vi "FV-resample-split_water.vi"(5 "Max Frequency":dbl, 7 "min Frequency":dbl, 10 "water":T1) -> (2 "water out":T1)   [LabVIEW 2020, in "FV-file_viewer.lvlib"]
uses:
  FV-file_viewer.lvlib
  FV-water_cluster.ctl
  FV-single_XY_plot.ctl
panel:
  out "Position":i32
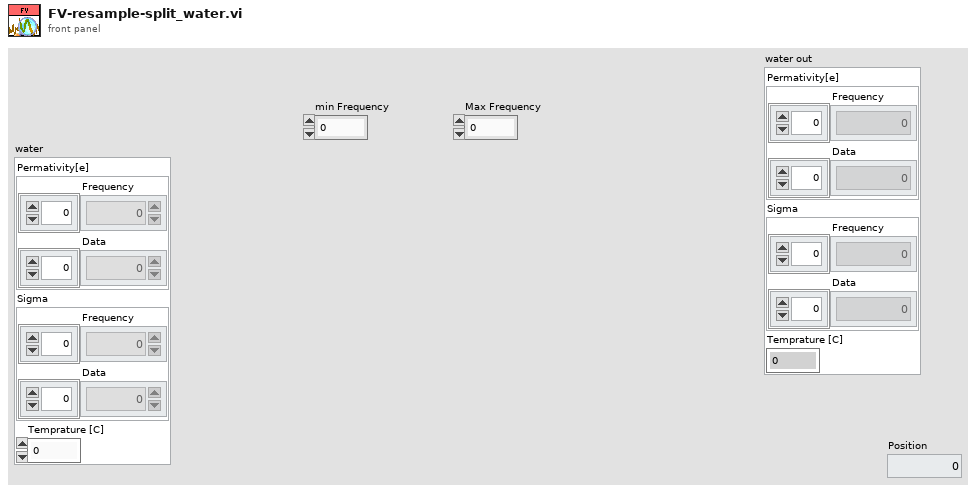
[diagram p1: front panel]
types:
  T1 = typedef "FV-file_viewer.lvlib/FV-water_cluster.ctl" = cluster{"Permativity[e]":T2, "Sigma":T2, "Temprature [C]":dbl}
  T2 = typedef "FV-file_viewer.lvlib/FV-single_XY_plot.ctl" = cluster{"Frequency":dbl[], "Data":dbl[]}
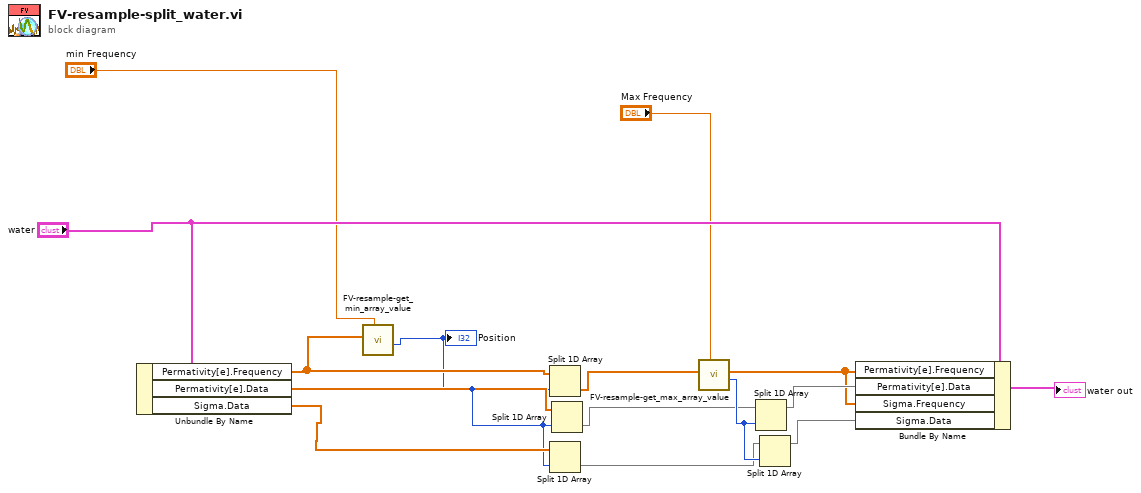
[diagram p0: block diagram]
diagram:
  n1 = Unbundle By Name("water") -> ("Permativity[e].Frequency"=w3:dbl[], "Permativity[e].Data"=w9:dbl[], "Sigma.Data"=w8:dbl[])
  n2 = call "FV-resample-get_min_array_value.vi"("min Frequency"="min Frequency", "Frequency array"=w3) -> ("Position"=w1:i32)  [unwired: 9 in]
  "Position" <- w1
  n3 = Split 1D Array(array=w3, index=w1) -> (second subarray=w7:dbl[])  [unwired: 1 out]
  n4 = Split 1D Array(array=w8, index=w1) -> (second subarray=w5:dbl[])  [unwired: 1 out]
  n5 = Split 1D Array(array=w9, index=w1) -> (second subarray=w6:dbl[])  [unwired: 1 out]
  n6 = call "FV-resample-get_max_array_value.vi"("max Frequency"="Max Frequency", "Frequency array"=w7) -> ("Position"=w12:i32, "cut array"=w4:dbl[])  [unwired: 8 in]
  n7 = Split 1D Array(array=w6, index=w12) -> (first subarray=w11:dbl[])  [unwired: 1 out]
  n8 = Split 1D Array(array=w5, index=w12) -> (first subarray=w10:dbl[])  [unwired: 1 out]
  n9 = Bundle By Name(cluster="water", "Permativity[e].Frequency"=w4, "Permativity[e].Data"=w11, "Sigma.Frequency"=w4, "Sigma.Data"=w10) -> (→"water out":T1)
